vi "New Explorer Hat Pro.vi"(8 "error in (no error)":errorcluster, 11 "LINX Resource":T1={"IO"=enum."Remote", "Interface"=enum."Serial", "LINX Device Config"={"Interface"=enum."Serial", "COM Port"="COM13", "TCP Configuration"={"IP Address"="", "Port"=0}, "Device Family"=1, "Device ID"=1, "Device Name"="myRIO-1900", "TCP Ref"=refnum, "Channels"={"DI"=[0, 1, 2, 3, 4, 5, 6, 7, 8, 9, 10, 11, 12, 13, 14, 15, 16, 17, 18, 19, 20, 21, 22, 23, 24, 25, 26, 27, 28, 29, 30, 31, 32, 33, 34, 35, 36, 37, 38, 39, 40, 41, 42, 43, 44, 45, 46], "DO"=[0, 1, 2, 3, 4, 5, 6, 7, 8, 9, 10, 11, 12, 13, 14, 15, 16, 17, 18, 19, 20, 21, 22, 23, 24, 25, 26, 27, 28, 29, 30, 31, 32, 33, 34, 35, 36, 37, 38, 39, 40, 41, 42, 43, 44, 45, 46], "AI"=[0, 1, 2, 3, 4, 5, 6, 7, 8, 9, 10, 11], "AO"=[], "PWM"=[3, 5, 6, 9, 10], "QE"=[], "UART"=[0, 1], "I2C 2"=[0], "SPI"=[0], "CAN"=[], "Servo"=[], "AI Ref (V)"=0.0, "AI Resolution (Bits)"=0, "AO Ref (V)"=0.0, "AO Resolution (Bits)"=0}}}) -> (0 "error out":errorcluster, 3 "ExplorerHatPro out":refnum<class "LINX-ExplorerHatPro.lvclass">)   [LabVIEW 2020, in "LINX-ExplorerHatPro.lvclass"]
uses:
  LINX-ExplorerHatPro.lvclass
  <vilib>/MakerHub/LINX/Private/Type Defs/LINX Ref.ctl
  <vilib>/MakerHub/LINX/Private/Type Defs/Platform.ctl
  <vilib>/MakerHub/LINX/Private/Type Defs/Interface.ctl
  <vilib>/MakerHub/LINX/Private/Device/Type Defs/LINX Device Config.ctl
  <vilib>/MakerHub/LINX/Private/Device/Type Defs/TCP Config.ctl
  <vilib>/MakerHub/LINX/Private/Device/Type Defs/Channels.ctl
  LINX-ADS1015/ADC Type Selection.ctl
  LINX-ExplorerHatPro.lvclass/LINX-ExplorerHatPro.ctl
  Write GPIO.vi
  Write ADS1015.vi
  LINX I2C/LINX I2C.lvclass
  GPIO/LINX GPIO.lvclass
  LINX-ADS1015/LINX-ADS1X15.lvclass
  CAP1208/CAP1208.lvclass
  <vilib>/MakerHub/LINX/LMH-LINX.lvlib
  <vilib>/MakerHub/LINX/Private/Device/Device.lvlib
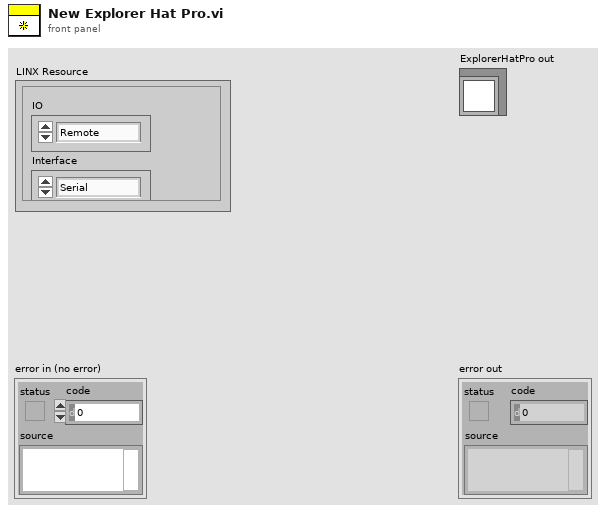
[diagram p1: front panel]
types:
  T1 = typedef "LMH-LINX.lvlib/LINX Ref.ctl" = cluster{"IO":T2, "Interface":T3, "LINX Device Config":T4}
  T2 = typedef "LMH-LINX.lvlib/Platform.ctl" = enum16{"Remote", "Local"}
  T3 = typedef "LMH-LINX.lvlib/Interface.ctl" = enum16{"Serial", "TCP"}
  T4 = typedef "LMH-LINX.lvlib/Device.lvlib/LINX Device Config.ctl" = cluster{"Interface":T3, "COM Port":refnum<visa-resource-name>, "TCP Configuration":T5, "Device Family":u8, "Device ID":u8, "Device Name":string, "TCP Ref":refnum<k5>, "Channels":T6}
  T5 = typedef "LMH-LINX.lvlib/Device.lvlib/TCP Config.ctl" = cluster{"IP Address":string, "Port":u16}
  T6 = typedef "LMH-LINX.lvlib/Channels.ctl" = cluster{"DI":u8[], "DO":u8[], "AI":u8[], "AO":u8[], "PWM":u8[], "QE":u8[], "UART":u8[], "I2C 2":u8[], "SPI":u8[], "CAN":u8[], "Servo":u8[], "AI Ref (V)":dbl, "AI Resolution (Bits)":u8, "AO Ref (V)":dbl, "AO Resolution (Bits)":u8}
  T7 = typedef "LINX-ADS1X15.lvclass/ADC Type Selection.ctl" = enum16{"ADS1015", "ADS1115"}
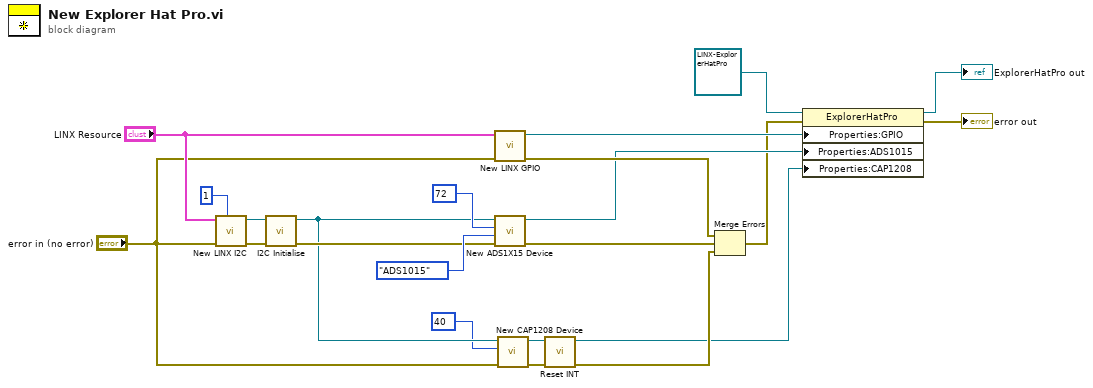
[diagram p0: block diagram]
diagram:
  n1 = call "New LINX I2C.vi"("LINX I2C Channel"=u8 1, "error in (no error)"="error in (no error)", "LINX Resource"="LINX Resource") -> ("error out"=w20:errorcluster, "LINX I2C out"=w19:refnum<class "LINX I2C.lvclass">)  [unwired: 7 in]
  n2 = call-dynamic "I2C Initialise.vi"("error in (no error)"=w20, "LINX I2C in"=w19) -> ("error out"=w18:errorcluster, "LINX I2C out"=w7:refnum<class "LINX I2C.lvclass">)  [unwired: 8 in]
  n3 = call "New LINX GPIO.vi"("error in (no error)"="error in (no error)", "LINX Resource"="LINX Resource") -> ("error out"=w13:errorcluster, "GPIO out"=w12:refnum<class "LINX GPIO.lvclass">)  [unwired: 8 in]
  n4 = call "New ADS1X15 Device.vi"("error in (no error)"=w18, "ADC Type (ADS1015)"=ADC_Type_Selection."ADS1015", "I2C Slave Address (0x48)"=u8 72, "I2C"=w7) -> ("error out"=w14:errorcluster, "LINX-ADS1X15 out"=w11:refnum<class "LINX-ADS1X15.lvclass">)  [unwired: 6 in]
  n5 = call "New CAP1208 Device.vi"("error in (no error)"="error in (no error)", "I2C Slave Address (0x28)"=u8 40, "I2C"=w7) -> ("error out"=w3:errorcluster, "CAP1208 out"=w4:refnum<class "CAP1208.lvclass">)  [unwired: 7 in]
  n6 = call "Reset INT.vi"("error in (no error)"=w3, "CAP1208 in"=w4) -> ("error out"=w2:errorcluster, "CAP1208 out"=w1:refnum<class "CAP1208.lvclass">)  [unwired: 8 in]
  n7 = Merge Errors(w13, w14, w2) -> (w10:errorcluster)
  n8 = property class="ExplorerHatPro"(reference=refnum<class "LINX-ExplorerHatPro.lvclass"> refnum ("ExplorerHatPro in"), error in=w10, "Properties:GPIO"=w12, "Properties:ADS1015"=w11, "Properties:CAP1208"=w1) -> (reference out=→"ExplorerHatPro out":refnum<class "LINX-ExplorerHatPro.lvclass">, error out=→"error out":errorcluster)
